vi "Set Cell Value (Error).vi"(8 "error in":errorcluster, 9 "Value":errorcluster, 10 "Cell Address":string, 11 "Worksheet in":refnum<k24>) -> (0 "error out":errorcluster, 3 "Worksheet out":refnum<k24>)   [LabVIEW 2019, in "Open Xml.lvlib"]
uses:
  Open Xml.lvlib
  D:/git/Open-Xml-LabVIEW/Source/DocumentFormat.OpenXml.dll
  DocumentFormat.OpenXml.dll
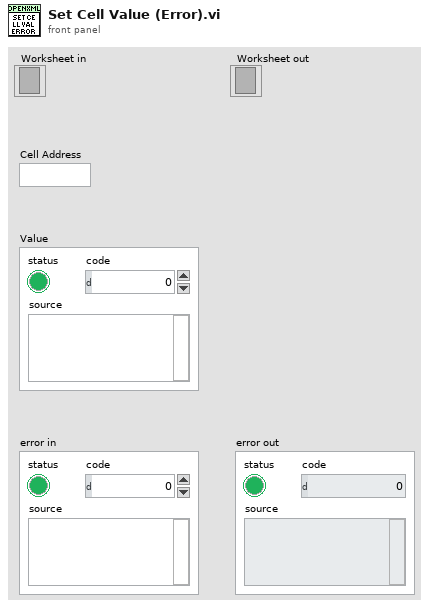
[diagram p1: front panel]
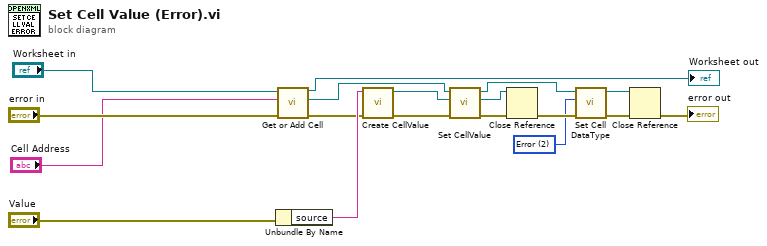
[diagram p0: block diagram]
diagram:
  w8 = 2 items=["Boolean", "Number", "Error", "SharedString", "String", "InlineString", "Date"] ("Datatype")
  n1 = Unbundle By Name("Value") -> ("source"=w13:string)
  n2 = call "Get or Add Cell.vi"("error in"="error in", "Cell Address"="Cell Address", "Worksheet in"="Worksheet in") -> ("error out"=w3:errorcluster, "Cell"=w10:refnum<k24>, "Worksheet out"=→"Worksheet out":refnum<k24>)  [unwired: 6 in]
  n3 = call "Create CellValue.vi"("error in"=w3, "Text"=w13) -> ("error out"=w4:errorcluster, "CellValue out"=w9:refnum<k24>)  [unwired: 8 in]
  n4 = call "Set CellValue.vi"("error in"=w4, "CellValue in"=w9, "Cell in"=w10) -> ("error out"=w7:errorcluster, "CellValue out"=w15:refnum<k24>, "Cell out"=w6:refnum<k24>)  [unwired: 6 in]
  n5 = Close Reference(reference=w15, error in (no error)=w7) -> (error out=w14:errorcluster)
  n6 = call "Set Cell DataType.vi"("error in"=w14, "Datatype"=w8, "Cell in"=w6) -> ("error out"=w5:errorcluster, "Cell out"=w18:refnum<k24>)  [unwired: 7 in]
  n7 = Close Reference(reference=w18, error in (no error)=w5) -> (error out=→"error out":errorcluster)
